vi "List SNS Topics in Region.vi"() -> ()   [LabVIEW 2015]
doc: "Demonstrates how to list all Amazon SNS topics created by an authenticated user."
uses:
  Core/HTTP Request/Region.ctl
  Core/HTTP Request/AWS Credentials.ctl
  Core/ARN/ARN.lvclass/ARN.ctl
  Core/ARN/Read ARN.vi
  SNS/Topic/Topic.lvclass
  Core/HTTP Request/HTTP Request.lvclass
panel:
  out "Topics":i32(listbox)
  in  "Region":T1
  in  "Secret Key":string
  in  "Access Key":string
  # "Overview: Demonstrates how to list all Amazon SNS topics created by an authenticated user.\nRequirements: NI Cloud Toolkit for AWS and a registered Amazon AWS account\nInstructions:\n1. Specify the Access Key and Secret Key for your AWS account. You can create an account at http://aws.amazon.com.\n2. Specify a Phone Number for sending an SMS message. Note that the number must be in +1xxxyyyzzzz format.\n3. Run the VI. All the topics associated with your account should be listed in the Topics indicator."
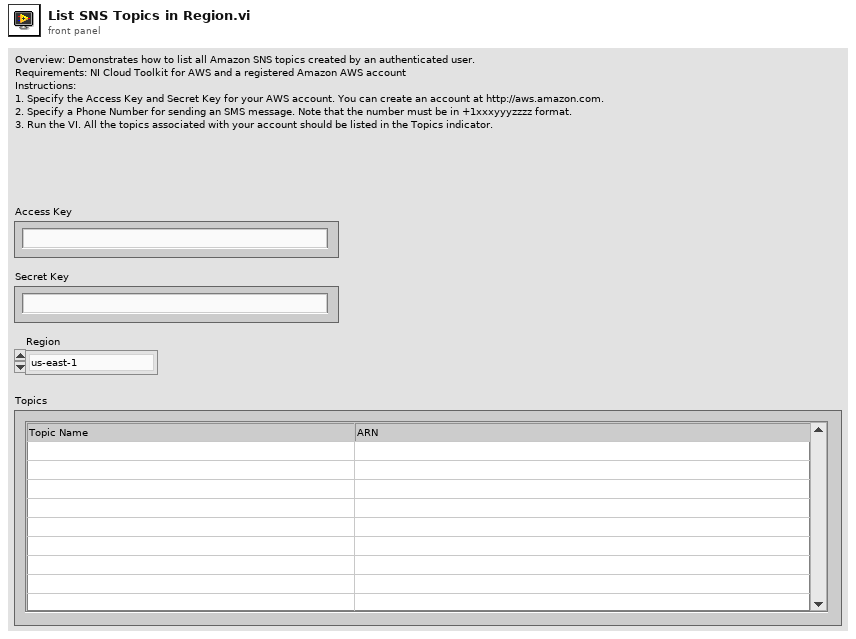
[diagram p1: front panel]
types:
  T1 = typedef "NI_AWS_Core.lvlib/HTTP Request.lvclass/Region.ctl" = enum16{"us-east-1", "us-east-2", "us-west-1", "us-west-2", "ap-northeast-1", "ap-northeast-2", "ap-southeast-1", "ap-southeast-2", "ca-central-1", "eu-central-1", "eu-west-1", "eu-west-2", "sa-east-1"}
  T2 = typedef "NI_AWS_Core.lvlib/HTTP Request.lvclass/AWS Credentials.ctl" = cluster{"Access Key":string, "Secret Key":string}
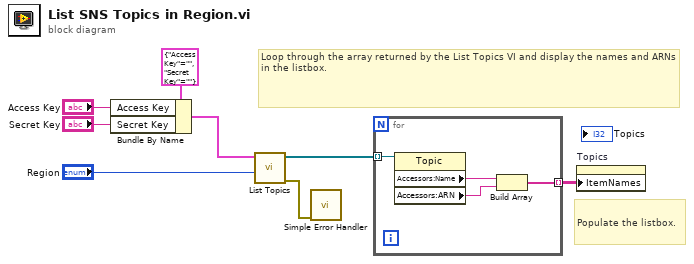
[diagram p0: block diagram]
diagram:
  # "Populate the listbox."
  # "Loop through the array returned by the List Topics VI and display the names and ARNs in the listbox."
  n1 = Bundle By Name(cluster=T2 {"Access Key"="", "Secret Key"=""} ("AWS Credentials"), "Access Key"="Access Key", "Secret Key"="Secret Key") -> (w5:T2)
  n2 = call "List Topics.vi"("Region"="Region", "AWS Credentials"=w5) -> ("error out"=w3:errorcluster, "Topics out"=w2:refnum<class "Topic.lvclass">[])  [unwired: 8 in]
  n3 = call <vilib>:"Simple Error Handler.vi"("error in (no error)"=w3) -> ()  [unwired: 4 in, 5 out]
  n4 = for {
    tunnel: w2 -> [w12] mode=indexing
    tunnel: [w9] -> w1 mode=indexing
    n5 = property class="Topic"(reference=w12) -> ("Accessors:Name"=w11:string, "Accessors:ARN"=w10:string)  [unwired: 1 in, 2 out]
    n6 = Build Array(w11, w10) -> (w9:string[])
  }
  n7 = property on="Topics" class="MCListbox (strict)"("ItemNames"=w1) -> ()  [unwired: 2 in, 2 out]
